vi "PH_Tektronix_7000.ProcCases.vi"(0 "i ref in":refnum<vi>, 1 "selector":string, 2 "Data":T4, 3 "call cluster":T5={"Object"="", "Selector"="", "CallType"=enum."synchronous", "Async Object"="", "Async Selector"="", "Data Descriptor"="", "Data"=[], "Error #"=0, "Expire"=0}, 5 "error in (no error)":errorcluster) -> (14 "i ref out":refnum<vi>, 17 "answer cluster":T5={"Object"="", "Selector"="", "CallType"=enum."synchronous", "Async Object"="", "Async Selector"="", "Data Descriptor"="", "Data"=[], "Error #"=0, "Expire"=0}, 19 "error out":errorcluster)   [LabVIEW 2014, in "PH_Tektronix_7000.lvlib"]
doc: "This method is called by a process from within the default case in the event loop. The methods of a class that are linked to events will be called from THIS method. Add your code here."
uses:
  PH_Tektronix_7000.lvlib
  CSCore/CSSystem/CoreDefs/CoreDefs.call_type.ctl
  CSCore/BaseProcess/BaseProcess.descriptor string definition.ctl
  CSCore/CSSystem/CoreDefs/CoreDefs.rawDataType.ctl
  PH_Tektronix_7000.Channel Config.ctl
  PH_Tektronix_7000.Trigger Config.ctl
  PH_Tektronix_7000.Acquisition Config.ctl
  CSCore/CSSystem/CoreLib/CoreLib.string 2 byte array.vi
  CSCore/CSSystem/CoreLib/CoreLib.byte array 2 short.vi
  CSCore/CSSystem/CoreLib/CoreLib.byte array 2 double.vi
  CSCore/CSSystem/CoreLib/CoreLib.byte array 2 string.vi
  CSCore/CSSystem/CoreLib/CoreLib.byte array 2 int.vi
  CSCore/BaseProcess/BaseProcess.lvlib
  CSCore/CSSystem/CoreLib/CoreLib.lvlib
  PH_PSDBWriter/PH_PSDBWriter.lvlib
  CSCore/CAEObj/CAEObj.lvlib
  CSCore/CSSystem/CSSystemLib/CSSystemLib.lvlib
panel:
  in  "Acqu Config":T1={"Record Length"=0, "Timebase [s/div]"=10000.0, "Position [%]"=0.0, "Acquisition Type"=1, "Average Waveforms"=10, "Envelope Waveforms"=10, "WfmDB Samples"=16000, "Continuous?"=FALSE, "Delay [s]"=0.0, "Run?"=FALSE} {"Delay [s]" format="%#_12p"; "Acquisition Type" items=["Sample", "Peak Detect", "Hi Res", "Average", "Envelope", "WfmDB"]; "Timebase [s/div]" format="%#_12g"}
  in  "Trig Config":T2 {"Trigger Mode" items=["Normal", "Auto"]; "Coupling" items=["DC", "AC", "Hf Reject", "Lf Reject", "Noise Rej", "Atrigger"]; "Slope" items=["Rise", "Fall", "Either"]; "Source" items=["Channel1"=0, "Channel2"=1, "Channel3"=2, "Channel4"=3, "Aux"=12, "Line"=13]}
  in  "Channel Config":T3={"Enable Channel"=FALSE, "Bandwidth"=0, "Input Impedance"=0, "Vertical Coupling"=0, "Probe Attenuation"=1.0, "Range [V/div]"=1.0, "Position [div]"=10.0, "Bandwidth raw"=""} {"Vertical Coupling" items=["AC", "DC", "Ground"]; "Input Impedance" items=["1M", "50"]; "Bandwidth" items=["FULL", "500 MHz", "250 MHz", "150 MHz", "20 MHz"]}
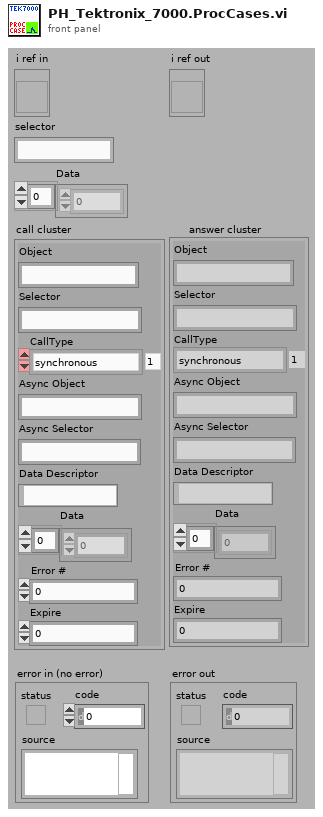
[diagram p1: front panel]
types:
  T1 = typedef "PH_Tektronix_7000.lvlib/PH_Tektronix_7000.Acquisition Config.ctl" = cluster{"Record Length":u32, "Timebase [s/div]":dbl, "Position [%]":dbl, "Acquisition Type":u16, "Average Waveforms":i32, "Envelope Waveforms":i32, "WfmDB Samples":i32, "Continuous?":bool, "Delay [s]":dbl, "Run?":bool}
  T2 = typedef "PH_Tektronix_7000.lvlib/PH_Tektronix_7000.Trigger Config.ctl" = cluster{"Source":u16, "Level [V]":dbl, "Slope":u16, "Coupling":u16, "Trigger Mode":u16}
  T3 = typedef "PH_Tektronix_7000.lvlib/PH_Tektronix_7000.Channel Config.ctl" = cluster{"Enable Channel":bool, "Bandwidth":u16, "Input Impedance":u16, "Vertical Coupling":u16, "Probe Attenuation":dbl, "Range [V/div]":dbl, "Position [div]":dbl, "Bandwidth raw":string}
  T4 = typedef "CoreDefs.rawDataType.ctl" = i8[]
  T5 = typedef "CoreDefs.call_type.ctl" = cluster{"Object":string, "Selector":string, "CallType":enum16{"simple", "synchronous", "asynchronous"}, "Async Object":string, "Async Selector":string, "Data Descriptor":T6, "Data":T4, "Error #":i32, "Expire":u32}
  T6 = typedef "BaseProcess.lvlib/BaseProcess.descriptor string definition.ctl" = string
  T7 = typedef "PH_PSDBWriter.lvlib/PH_PSDBWriter.PHELIX-Subsystems.ctl" = i32
  T8 = typedef "PH_Tektronix_7000.lvlib/PH_Tektronix_7000.i attribute.ctl" = cluster{"VISA Resource Name":refnum<visa-resource-name>, "IDN":cluster{"Instrument Driver":string, "Instrument Firmware":string, "Model":string, "Serial Number":string}, "Selftest":cluster{"Result":i32, "Message":string}, "Trigger Configuration":T2, "Acquisition Configuration":T1, "GUI Refs":T9, "State":T10, "Error Message":string, "Allow Prdc Loop?":bool, "Channel 1":T3, "Channel 2":T3, "Channel 3":T3, "Channel 4":T3, "Data CH 1":waveform(dbl), "Data CH 2":waveform(dbl), "Data CH 3":waveform(dbl), "Data CH 4":waveform(dbl), "Allow config?":bool, "Name Channel 1":string, "Name Channel 2":string, "Name Channel 3":string, "Name Channel 4":string, "Fetch Data before sending to PSDB?":bool, "Constructor passed?":bool, "Data taken at":timestamp, "Plot Colors":u32[], "Default VISA Resource":string}
  T9 = typedef "PH_Tektronix_7000.lvlib/PH_Tektronix_7000.GUI Refs.ctl" = cluster{"Graph":refnum<vi>, "State":refnum<vi>, "Delete":refnum<vi>, "VISA Resource":refnum<vi>, "Allow Configure":refnum<vi>, "Fetch Data":refnum<vi>, "Fetch before sending Data to PSDB":refnum<vi>, "Name Channel 1":refnum<vi>, "Name Channel 2":refnum<vi>, "Name Channel 3":refnum<vi>, "Name Channel 4":refnum<vi>, "Prdc Intervall [ms]":refnum<vi>, "Data taken":refnum<vi>, "Model":refnum<vi>, "Serial Number":refnum<vi>, "Firmware":refnum<vi>, "Driver":refnum<vi>, "Acquisition":refnum<vi>, "Trigger":refnum<vi>, "Cursor: D Time [s]":refnum<vi>, "Cursor: D Signal [V]":refnum<vi>, "Channel 1":refnum<vi>, "Channel 2":refnum<vi>, "Channel 3":refnum<vi>, "Channel 4":refnum<vi>}
  T10 = typedef "PH_StatusHandler.lvlib/PH_StatusHandler.Status.ctl" = i16
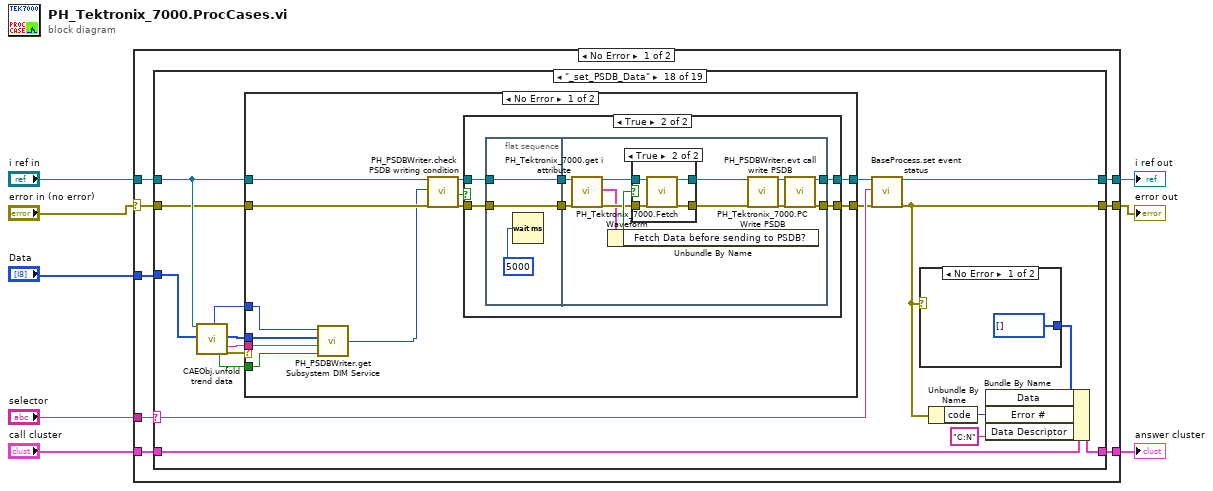
[diagram p0: block diagram]
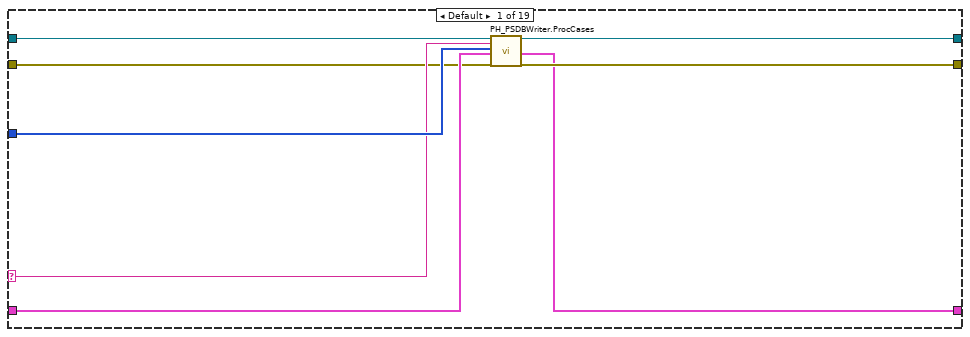
[diagram p2: hidden frame]
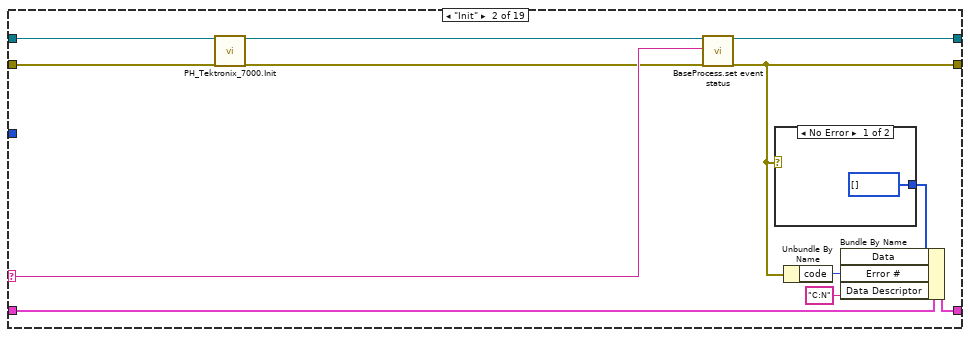
[diagram p3: hidden frame]
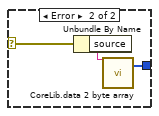
[diagram p4: hidden frame]
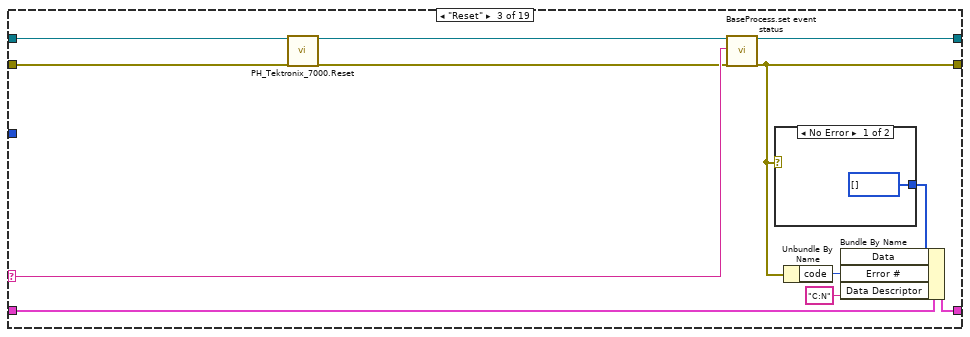
[diagram p5: hidden frame]
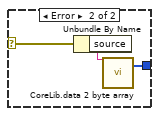
[diagram p6: hidden frame]
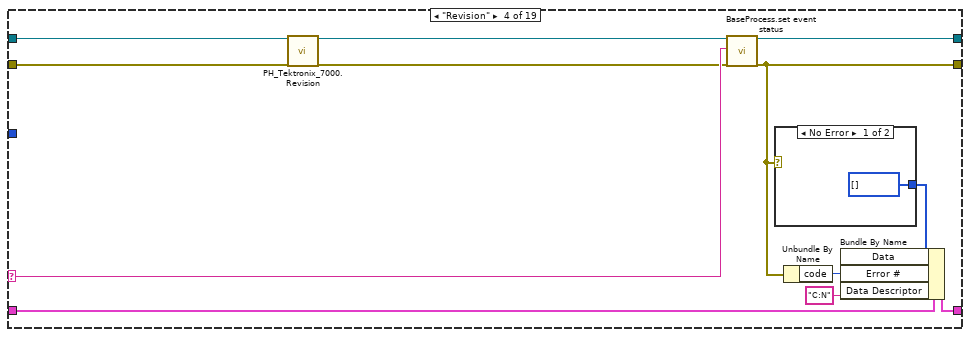
[diagram p7: hidden frame]
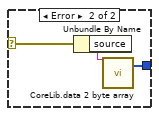
[diagram p8: hidden frame]
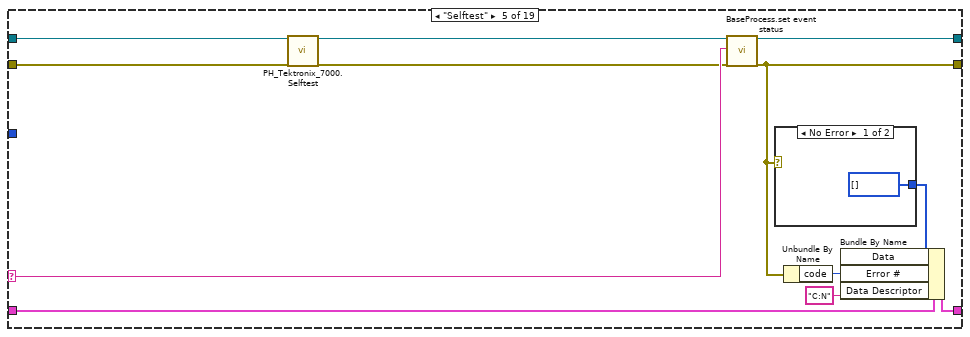
[diagram p9: hidden frame]
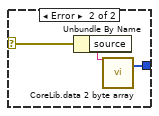
[diagram p10: hidden frame]
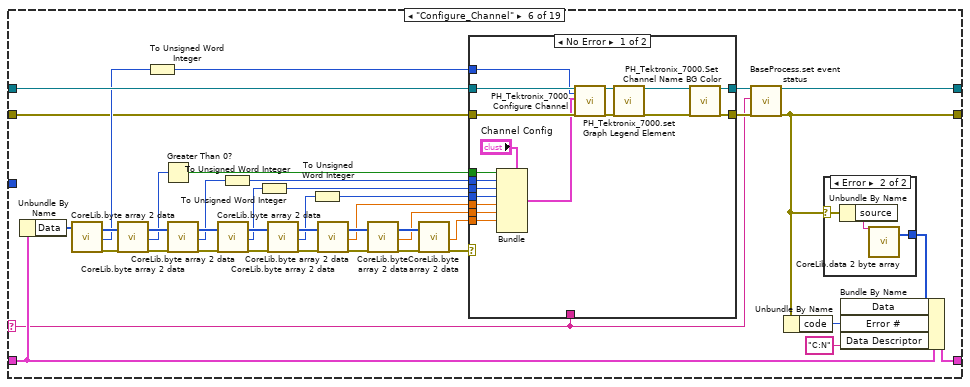
[diagram p11: hidden frame]
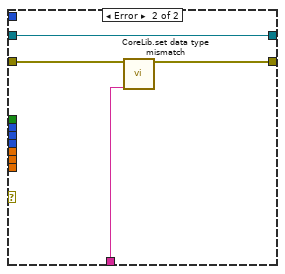
[diagram p12: hidden frame]
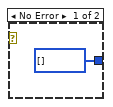
[diagram p13: hidden frame]
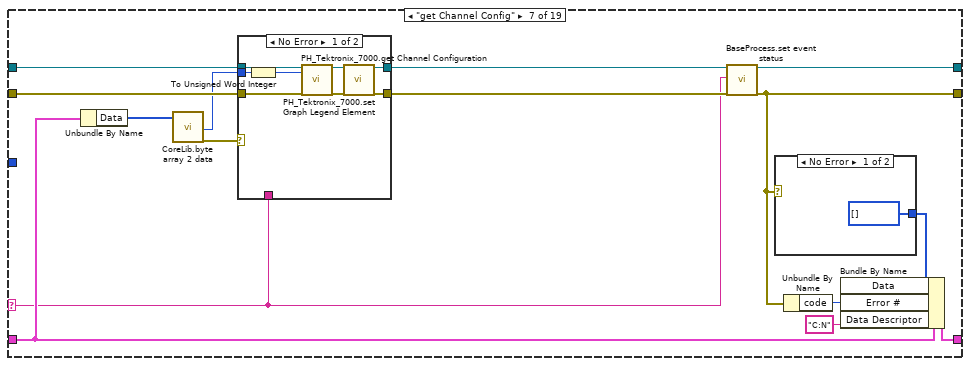
[diagram p14: hidden frame]
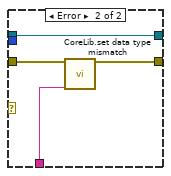
[diagram p15: hidden frame]
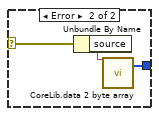
[diagram p16: hidden frame]
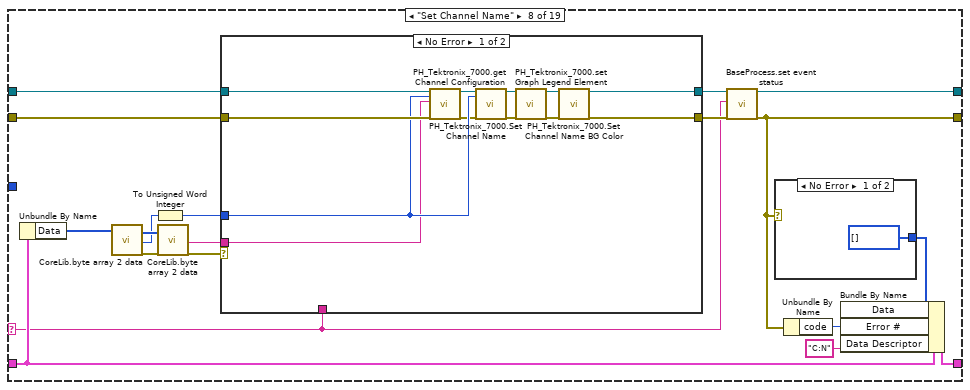
[diagram p17: hidden frame]
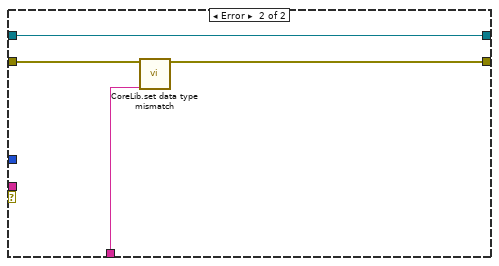
[diagram p18: hidden frame]
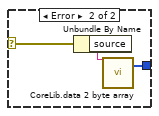
[diagram p19: hidden frame]
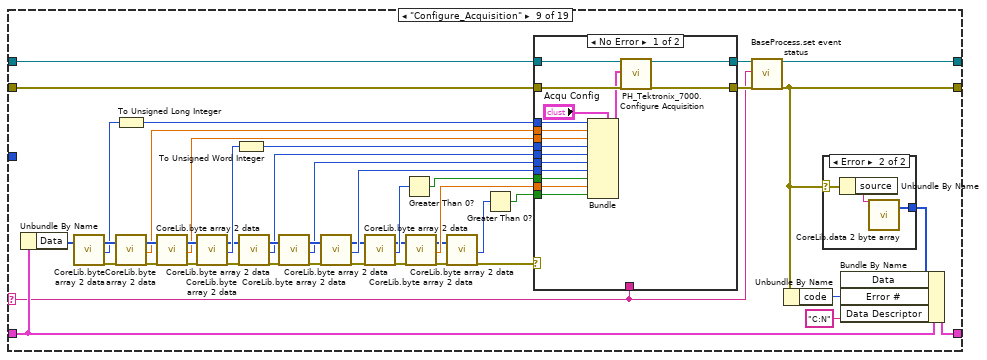
[diagram p20: hidden frame]
diagram:
  n1 = case shown="No Error" "error in (no error)" {
    selector: "error in (no error)" -> [w9 w614]
    tunnel: "selector" -> [w16 _]
    tunnel: [w15 w615] -> w7
    tunnel: "Data" -> [w14 _]
    tunnel: "call cluster" -> [w13 w615]
    tunnel: "i ref in" -> [w12 w616]
    tunnel: [w11 w616] -> w3
    tunnel: [w10 w614] -> w2
    frame No Error {
      n2 = case shown="\"_set_PSDB_Data\"" w16 {
        selector: w16 -> [w19 w29 w45 w61 w77 w100 w156 w192 w252 w297 w324 w363 w379 w394 w423 w464 w494 w543 w602]
        tunnel: w14 -> [w20 _ _ _ _ _ _ _ _ _ _ _ _ _ _ _ _ w533 _]
        tunnel: w12 -> [w18 w28 w44 w60 w76 w123 w164 w199 w265 w301 w336 w367 w383 w400 w429 w470 w499 w537 w601]
        tunnel: [w24 w32 w48 w64 w80 w125 w166 w201 w267 w303 w338 w369 w385 w405 w434 w475 w503 w546 w605] -> w11
        tunnel: w13 -> [w21 w30 w46 w62 w78 w120 w159 w196 w261 w298 w332 w364 w380 w398 w427 w468 w497 w544 w603]
        tunnel: [w22 w35 w51 w67 w83 w128 w169 w204 w270 w306 w341 w372 w388 w408 w437 w478 w506 w549 w608] -> w15
        tunnel: w9 -> [w17 w27 w43 w59 w75 w98 w161 w191 w251 w296 w323 w362 w378 w397 w426 w467 w496 w536 w599]
        tunnel: [w23 w33 w49 w65 w81 w126 w167 w202 w268 w304 w339 w370 w386 w406 w435 w476 w504 w547 w606] -> w10
        frame Default {
          n3 = call "PH_PSDBWriter.ProcCases.vi"("i ref in"=w18, "selector"=w19, "Data"=w20, "call cluster"=w21, "error in"=w17) -> ("i ref out"=w24:refnum<vi>, "answer cluster"=w22:T5, "error out"=w23:errorcluster)  [unwired: 12 in]
        }
        frame "Init" {
          n4 = call "PH_Tektronix_7000.Init.vi"("i ref in"=w28, "error in (no error)"=w27) -> ("i ref out"=w26:refnum<vi>, "error out"=w25:errorcluster)  [unwired: 16 in]
          n5 = call "BaseProcess.set event status.vi"("i ref in"=w26, "EventStatus"=w29, "error in (no error)"=w25) -> ("i ref out"=w32:refnum<vi>, "error out"=w33:errorcluster)  [unwired: 14 in, 1 out]
          n6 = case shown="No Error" w33 {
            selector: w33 -> [_ w40]
            tunnel: [T4 [] ("byteArray out") w39] -> w34
            frame No Error {
            }
            frame Error {
              n7 = Unbundle By Name(w40) -> ("source"=w38:string)
              n8 = call-poly "CoreLib.data 2 byte array.vi"("string"=w38) -> ("byteArray out"=w39:T4)  [unwired: 18 in]
            }
          }
          n9 = Unbundle By Name(w33) -> ("code"=w36:i32)
          n10 = Bundle By Name(cluster=w30, "Data"=w34, "Error #"=w36, "Data Descriptor"="C:N") -> (w35:T5)
        }
        frame "Reset" {
          n11 = call "PH_Tektronix_7000.Reset.vi"("i ref in"=w44, "error IO"=w43) -> ("i ref out"=w41:refnum<vi>, "error out"=w42:errorcluster)  [unwired: 16 in]
          n12 = call "BaseProcess.set event status.vi"("i ref in"=w41, "EventStatus"=w45, "error in (no error)"=w42) -> ("i ref out"=w48:refnum<vi>, "error out"=w49:errorcluster)  [unwired: 14 in, 1 out]
          n13 = case shown="No Error" w49 {
            selector: w49 -> [_ w56]
            tunnel: [T4 [] ("byteArray out") w55] -> w50
            frame No Error {
            }
            frame Error {
              n14 = Unbundle By Name(w56) -> ("source"=w54:string)
              n15 = call-poly "CoreLib.data 2 byte array.vi"("string"=w54) -> ("byteArray out"=w55:T4)  [unwired: 18 in]
            }
          }
          n16 = Unbundle By Name(w49) -> ("code"=w52:i32)
          n17 = Bundle By Name(cluster=w46, "Data"=w50, "Error #"=w52, "Data Descriptor"="C:N") -> (w51:T5)
        }
        frame "Revision" {
          n18 = call "PH_Tektronix_7000.Revision.vi"("i ref in"=w60, "error IO"=w59) -> ("i ref out"=w57:refnum<vi>, "error out"=w58:errorcluster)  [unwired: 16 in]
          n19 = call "BaseProcess.set event status.vi"("i ref in"=w57, "EventStatus"=w61, "error in (no error)"=w58) -> ("i ref out"=w64:refnum<vi>, "error out"=w65:errorcluster)  [unwired: 14 in, 1 out]
          n20 = case shown="No Error" w65 {
            selector: w65 -> [_ w72]
            tunnel: [T4 [] ("byteArray out") w71] -> w66
            frame No Error {
            }
            frame Error {
              n21 = Unbundle By Name(w72) -> ("source"=w70:string)
              n22 = call-poly "CoreLib.data 2 byte array.vi"("string"=w70) -> ("byteArray out"=w71:T4)  [unwired: 18 in]
            }
          }
          n23 = Unbundle By Name(w65) -> ("code"=w68:i32)
          n24 = Bundle By Name(cluster=w62, "Data"=w66, "Error #"=w68, "Data Descriptor"="C:N") -> (w67:T5)
        }
        frame "Selftest" {
          n25 = call "PH_Tektronix_7000.Selftest.vi"("i ref in"=w76, "error IO"=w75) -> ("i ref out"=w73:refnum<vi>, "error out"=w74:errorcluster)  [unwired: 16 in]
          n26 = call "BaseProcess.set event status.vi"("i ref in"=w73, "EventStatus"=w77, "error in (no error)"=w74) -> ("i ref out"=w80:refnum<vi>, "error out"=w81:errorcluster)  [unwired: 14 in, 1 out]
          n27 = case shown="No Error" w81 {
            selector: w81 -> [_ w88]
            tunnel: [T4 [] ("byteArray out") w87] -> w82
            frame No Error {
            }
            frame Error {
              n28 = Unbundle By Name(w88) -> ("source"=w86:string)
              n29 = call-poly "CoreLib.data 2 byte array.vi"("string"=w86) -> ("byteArray out"=w87:T4)  [unwired: 18 in]
            }
          }
          n30 = Unbundle By Name(w81) -> ("code"=w84:i32)
          n31 = Bundle By Name(cluster=w78, "Data"=w82, "Error #"=w84, "Data Descriptor"="C:N") -> (w83:T5)
        }
        frame "Configure_Channel" {
          n32 = Unbundle By Name(w120) -> ("Data"=w90:T4)
          n33 = call-poly "CoreLib.byte array 2 data.vi"("byteArray"=w90) -> ("byteArray out"=w112:T4, "i16"=w105:i16, "error out"=w119:errorcluster)  [unwired: 16 in]
          n34 = call-poly "CoreLib.byte array 2 data.vi"("byteArray"=w112, "error in (no error)"=w119) -> ("byteArray out"=w111:T4, "i16"=w95:i16, "error out"=w118:errorcluster)  [unwired: 15 in]
          n35 = To Unsigned Word Integer(number=w105) -> (unsigned 16bit integer=w89:u16)
          n36 = Greater Than 0?(x=w95) -> (x > 0?=w94:bool)
          n37 = call-poly "CoreLib.byte array 2 data.vi"("byteArray"=w111, "error in (no error)"=w118) -> ("byteArray out"=w110:T4, "i16"=w104:i16, "error out"=w117:errorcluster)  [unwired: 15 in]
          n38 = call-poly "CoreLib.byte array 2 data.vi"("byteArray"=w110, "error in (no error)"=w117) -> ("byteArray out"=w109:T4, "i16"=w97:i16, "error out"=w116:errorcluster)  [unwired: 15 in]
          n39 = To Unsigned Word Integer(number=w104) -> (unsigned 16bit integer=w93:u16)
          n40 = To Unsigned Word Integer(number=w97) -> (unsigned 16bit integer=w92:u16)
          n41 = call-poly "CoreLib.byte array 2 data.vi"("byteArray"=w109, "error in (no error)"=w116) -> ("byteArray out"=w108:T4, "i16"=w96:i16, "error out"=w115:errorcluster)  [unwired: 15 in]
          n42 = To Unsigned Word Integer(number=w96) -> (unsigned 16bit integer=w91:u16)
          n43 = call-poly "CoreLib.byte array 2 data.vi"("byteArray"=w108, "error in (no error)"=w115) -> ("byteArray out"=w107:T4, "d64"=w103:dbl, "error out"=w114:errorcluster)  [unwired: 15 in]
          n44 = call-poly "CoreLib.byte array 2 data.vi"("byteArray"=w107, "error in (no error)"=w114) -> ("byteArray out"=w106:T4, "d64"=w102:dbl, "error out"=w113:errorcluster)  [unwired: 15 in]
          n45 = call-poly "CoreLib.byte array 2 data.vi"("byteArray"=w106, "error in (no error)"=w113) -> ("d64"=w101:dbl, "error out"=w99:errorcluster)  [unwired: 15 in, 1 out]
          n46 = case shown="No Error" w99 {
            tunnel: w123 -> [w147 w151]
            tunnel: [w132 w149] -> w122
            tunnel: [w130 w151] -> w121
            tunnel: w94 -> [w143 _]
            tunnel: w93 -> [w142 _]
            tunnel: w92 -> [w141 _]
            tunnel: w91 -> [w140 _]
            tunnel: w103 -> [w139 _]
            tunnel: w102 -> [w138 _]
            tunnel: w101 -> [w137 _]
            tunnel: w100 -> [_ w150]
            tunnel: w98 -> [w146 w148]
            tunnel: w89 -> [w136 _]
            frame No Error {
              n47 = Bundle(cluster="Channel Config", "Enable Channel"=w143, "Bandwidth"=w142, "Input Impedance"=w141, "Vertical Coupling"=w140, "Probe Attenuation"=w139, "Range [V/div]"=w138, "Position [div]"=w137) -> (w144:T3)  [unwired: 1 in]
              n48 = call "PH_Tektronix_7000.Configure Channel.vi"("i ref in"=w147, "Channel"=w136, "Channel Configuration"=w144, "error IO"=w146) -> ("i ref out"=w133:refnum<vi>, "error out"=w134:errorcluster)  [unwired: 14 in]
              n49 = call "PH_Tektronix_7000.set Graph Legend Element.vi"("i ref in"=w133, "error in (no error)"=w134) -> ("i ref out"=w131:refnum<vi>, "error out"=w135:errorcluster)  [unwired: 16 in]
              n50 = call "PH_Tektronix_7000.Set Channel Name BG Color.vi"("i ref in"=w131, "error in"=w135) -> ("i ref out"=w130:refnum<vi>, "error out"=w132:errorcluster)  [unwired: 16 in]
            }
            frame Error {
              n51 = call "CoreLib.set data type mismatch.vi"("error in (no error)"=w148, "error source"=w150) -> ("error out"=w149:errorcluster)  [unwired: 17 in]
            }
          }
          n52 = call "BaseProcess.set event status.vi"("i ref in"=w121, "EventStatus"=w100, "error in (no error)"=w122) -> ("i ref out"=w125:refnum<vi>, "error out"=w126:errorcluster)  [unwired: 14 in, 1 out]
          n53 = Unbundle By Name(w126) -> ("code"=w129:i32)
          n54 = case shown="Error" w126 {
            selector: w126 -> [_ w155]
            tunnel: [T4 [] ("byteArray out") w154] -> w127
            frame No Error {
            }
            frame Error {
              n55 = Unbundle By Name(w155) -> ("source"=w153:string)
              n56 = call-poly "CoreLib.data 2 byte array.vi"("string"=w153) -> ("byteArray out"=w154:T4)  [unwired: 18 in]
            }
          }
          n57 = Bundle By Name(cluster=w120, "Data"=w127, "Error #"=w129, "Data Descriptor"="C:N") -> (w128:T5)
        }
        frame "get Channel Config" {
          n58 = Unbundle By Name(w159) -> ("Data"=w160:T4)
          n59 = call-poly "CoreLib.byte array 2 data.vi"("byteArray"=w160) -> ("i16"=w158:i16, "error out"=w157:errorcluster)  [unwired: 16 in, 1 out]
          n60 = case shown="No Error" w157 {
            tunnel: w164 -> [w178 w180]
            tunnel: [w171 w181] -> w163
            tunnel: [w173 w180] -> w162
            tunnel: w161 -> [w177 w182]
            tunnel: w158 -> [w175 _]
            tunnel: w156 -> [_ w179]
            frame No Error {
              n61 = To Unsigned Word Integer(number=w175) -> (unsigned 16bit integer=w176:u16)
              n62 = call "PH_Tektronix_7000.get Channel Configuration.vi"("i ref in"=w178, "Channel"=w176, "error IO"=w177) -> ("i ref out"=w174:refnum<vi>, "error out"=w172:errorcluster)  [unwired: 15 in]
              n63 = call "PH_Tektronix_7000.set Graph Legend Element.vi"("i ref in"=w174, "error in (no error)"=w172) -> ("i ref out"=w173:refnum<vi>, "error out"=w171:errorcluster)  [unwired: 16 in]
            }
            frame Error {
              n64 = call "CoreLib.set data type mismatch.vi"("error in (no error)"=w182, "error source"=w179) -> ("error out"=w181:errorcluster)  [unwired: 17 in]
            }
          }
          n65 = call "BaseProcess.set event status.vi"("i ref in"=w162, "EventStatus"=w156, "error in (no error)"=w163) -> ("i ref out"=w166:refnum<vi>, "error out"=w167:errorcluster)  [unwired: 14 in, 1 out]
          n66 = case shown="No Error" w167 {
            selector: w167 -> [_ w186]
            tunnel: [T4 [] ("byteArray out") w185] -> w168
            frame No Error {
            }
            frame Error {
              n67 = Unbundle By Name(w186) -> ("source"=w184:string)
              n68 = call-poly "CoreLib.data 2 byte array.vi"("string"=w184) -> ("byteArray out"=w185:T4)  [unwired: 18 in]
            }
          }
          n69 = Unbundle By Name(w167) -> ("code"=w170:i32)
          n70 = Bundle By Name(cluster=w159, "Data"=w168, "Error #"=w170, "Data Descriptor"="C:N") -> (w169:T5)
        }
        frame "Set Channel Name" {
          n71 = Unbundle By Name(w196) -> ("Data"=w190:T4)
          n72 = call-poly "CoreLib.byte array 2 data.vi"("byteArray"=w190) -> ("byteArray out"=w194:T4, "i16"=w193:i16, "error out"=w195:errorcluster)  [unwired: 16 in]
          n73 = To Unsigned Word Integer(number=w193) -> (unsigned 16bit integer=w189:u16)
          n74 = call-poly "CoreLib.byte array 2 data.vi"("byteArray"=w194, "error in (no error)"=w195) -> ("string"=w188:string, "error out"=w187:errorcluster)  [unwired: 15 in, 1 out]
          n75 = case shown="No Error" w187 {
            tunnel: w199 -> [w217 w221]
            tunnel: [w208 w219] -> w198
            tunnel: [w206 w221] -> w197
            tunnel: w192 -> [_ w220]
            tunnel: w191 -> [w216 w218]
            tunnel: w189 -> [w212 _]
            tunnel: w188 -> [w209 _]
            frame No Error {
              n76 = call "PH_Tektronix_7000.Set Channel Name.vi"("i ref in"=w217, "Channel"=w212, "Channel Name"=w209, "error IO"=w216) -> ("i ref out"=w211:refnum<vi>, "error out"=w210:errorcluster)  [unwired: 14 in]
              n77 = call "PH_Tektronix_7000.get Channel Configuration.vi"("i ref in"=w211, "Channel"=w212, "error IO"=w210) -> ("i ref out"=w215:refnum<vi>, "error out"=w214:errorcluster)  [unwired: 15 in]
              n78 = call "PH_Tektronix_7000.set Graph Legend Element.vi"("i ref in"=w215, "error in (no error)"=w214) -> ("i ref out"=w207:refnum<vi>, "error out"=w213:errorcluster)  [unwired: 16 in]
              n79 = call "PH_Tektronix_7000.Set Channel Name BG Color.vi"("i ref in"=w207, "error in"=w213) -> ("i ref out"=w206:refnum<vi>, "error out"=w208:errorcluster)  [unwired: 16 in]
            }
            frame Error {
              n80 = call "CoreLib.set data type mismatch.vi"("error in (no error)"=w218, "error source"=w220) -> ("error out"=w219:errorcluster)  [unwired: 17 in]
            }
          }
          n81 = call "BaseProcess.set event status.vi"("i ref in"=w197, "EventStatus"=w192, "error in (no error)"=w198) -> ("i ref out"=w201:refnum<vi>, "error out"=w202:errorcluster)  [unwired: 14 in, 1 out]
          n82 = case shown="No Error" w202 {
            selector: w202 -> [_ w225]
            tunnel: [T4 [] ("byteArray out") w224] -> w203
            frame No Error {
            }
            frame Error {
              n83 = Unbundle By Name(w225) -> ("source"=w223:string)
              n84 = call-poly "CoreLib.data 2 byte array.vi"("string"=w223) -> ("byteArray out"=w224:T4)  [unwired: 18 in]
            }
          }
          n85 = Unbundle By Name(w202) -> ("code"=w205:i32)
          n86 = Bundle By Name(cluster=w196, "Data"=w203, "Error #"=w205, "Data Descriptor"="C:N") -> (w204:T5)
        }
        frame "Configure_Acquisition" {
          n87 = Unbundle By Name(w261) -> ("Data"=w262:T4)
          n88 = call-poly "CoreLib.byte array 2 data.vi"("byteArray"=w262) -> ("byteArray out"=w257:T4, "i32"=w254:i32, "error out"=w260:errorcluster)  [unwired: 16 in]
          n89 = To Unsigned Long Integer(number=w254) -> (unsigned 32bit integer=w247:u32)
          n90 = call-poly "CoreLib.byte array 2 data.vi"("byteArray"=w257, "error in (no error)"=w260) -> ("byteArray out"=w256:T4, "d64"=w246:dbl, "error out"=w259:errorcluster)  [unwired: 15 in]
          n91 = call-poly "CoreLib.byte array 2 data.vi"("byteArray"=w256, "error in (no error)"=w259) -> ("byteArray out"=w255:T4, "d64"=w253:dbl, "error out"=w258:errorcluster)  [unwired: 15 in]
          n92 = call-poly "CoreLib.byte array 2 data.vi"("byteArray"=w255, "error in (no error)"=w258) -> ("byteArray out"=w240:T4, "i16"=w248:i16, "error out"=w239:errorcluster)  [unwired: 15 in]
          n93 = To Unsigned Word Integer(number=w248) -> (unsigned 16bit integer=w245:u16)
          n94 = call-poly "CoreLib.byte array 2 data.vi"("byteArray"=w240, "error in (no error)"=w239) -> ("byteArray out"=w242:T4, "i32"=w238:i32, "error out"=w244:errorcluster)  [unwired: 15 in]
          n95 = call-poly "CoreLib.byte array 2 data.vi"("byteArray"=w242, "error in (no error)"=w244) -> ("byteArray out"=w241:T4, "i32"=w237:i32, "error out"=w243:errorcluster)  [unwired: 15 in]
          n96 = call-poly "CoreLib.byte array 2 data.vi"("byteArray"=w241, "error in (no error)"=w243) -> ("byteArray out"=w226:T4, "i32"=w236:i32, "error out"=w229:errorcluster)  [unwired: 15 in]
          n97 = call-poly "CoreLib.byte array 2 data.vi"("byteArray"=w226, "error in (no error)"=w229) -> ("byteArray out"=w234:T4, "i16"=w250:i16, "error out"=w235:errorcluster)  [unwired: 15 in]
          n98 = Greater Than 0?(x=w250) -> (x > 0?=w249:bool)
          n99 = call-poly "CoreLib.byte array 2 data.vi"("byteArray"=w234, "error in (no error)"=w235) -> ("byteArray out"=w230:T4, "d64"=w233:dbl, "error out"=w232:errorcluster)  [unwired: 15 in]
          n100 = call-poly "CoreLib.byte array 2 data.vi"("byteArray"=w230, "error in (no error)"=w232) -> ("i16"=w228:i16, "error out"=w231:errorcluster)  [unwired: 15 in, 1 out]
          n101 = Greater Than 0?(x=w228) -> (x > 0?=w227:bool)
          n102 = case shown="No Error" w231 {
            tunnel: w265 -> [w287 w291]
            tunnel: [w272 w289] -> w264
            tunnel: [w273 w291] -> w263
            tunnel: w247 -> [w284 _]
            tunnel: w246 -> [w283 _]
            tunnel: w253 -> [w282 _]
            tunnel: w245 -> [w281 _]
            tunnel: w249 -> [w276 _]
            tunnel: w252 -> [_ w290]
            tunnel: w251 -> [w286 w288]
            tunnel: w238 -> [w279 _]
            tunnel: w237 -> [w278 _]
            tunnel: w236 -> [w277 _]
            tunnel: w233 -> [w275 _]
            tunnel: w227 -> [w274 _]
            frame No Error {
              n103 = Bundle(cluster="Acqu Config", "Record Length"=w284, "Timebase [s/div]"=w283, "Position [%]"=w282, "Acquisition Type"=w281, "Average Waveforms"=w279, "Envelope Waveforms"=w278, "WfmDB Samples"=w277, "Continuous?"=w276, "Delay [s]"=w275, "Run?"=w274) -> (w280:T1)
              n104 = call "PH_Tektronix_7000.Configure Acquisition.vi"("i ref in"=w287, "Acquisition Configuration"=w280, "error IO"=w286) -> ("i ref out"=w273:refnum<vi>, "error out"=w272:errorcluster)  [unwired: 15 in]
            }
            frame Error {
              n105 = call "CoreLib.set data type mismatch.vi"("error in (no error)"=w288, "error source"=w290) -> ("error out"=w289:errorcluster)  [unwired: 17 in]
            }
          }
          n106 = call "BaseProcess.set event status.vi"("i ref in"=w263, "EventStatus"=w252, "error in (no error)"=w264) -> ("i ref out"=w267:refnum<vi>, "error out"=w268:errorcluster)  [unwired: 14 in, 1 out]
          n107 = Unbundle By Name(w268) -> ("code"=w271:i32)
          n108 = case shown="Error" w268 {
            selector: w268 -> [_ w295]
            tunnel: [T4 [] ("byteArray out") w294] -> w269
            frame No Error {
            }
            frame Error {
              n109 = Unbundle By Name(w295) -> ("source"=w293:string)
              n110 = call-poly "CoreLib.data 2 byte array.vi"("string"=w293) -> ("byteArray out"=w294:T4)  [unwired: 18 in]
            }
          }
          n111 = Bundle By Name(cluster=w261, "Data"=w269, "Error #"=w271, "Data Descriptor"="C:N") -> (w270:T5)
        }
        frame "get Acquisition Config" {
          n112 = call "PH_Tektronix_7000.get Acquisition Configuration.vi"("i ref in"=w301, "error IO"=w296) -> ("i ref out"=w299:refnum<vi>, "error out"=w300:errorcluster)  [unwired: 16 in]
          n113 = call "BaseProcess.set event status.vi"("i ref in"=w299, "EventStatus"=w297, "error in (no error)"=w300) -> ("i ref out"=w303:refnum<vi>, "error out"=w304:errorcluster)  [unwired: 14 in, 1 out]
          n114 = case shown="No Error" w304 {
            selector: w304 -> [_ w311]
            tunnel: [T4 [] ("byteArray out") w310] -> w305
            frame No Error {
            }
            frame Error {
              n115 = Unbundle By Name(w311) -> ("source"=w309:string)
              n116 = call-poly "CoreLib.data 2 byte array.vi"("string"=w309) -> ("byteArray out"=w310:T4)  [unwired: 18 in]
            }
          }
          n117 = Unbundle By Name(w304) -> ("code"=w307:i32)
          n118 = Bundle By Name(cluster=w298, "Data"=w305, "Error #"=w307, "Data Descriptor"="C:N") -> (w306:T5)
        }
        frame "Configure_Trigger" {
          n119 = Unbundle By Name(w332) -> ("Data"=w333:T4)
          n120 = call-poly "CoreLib.byte array 2 data.vi"("byteArray"=w333) -> ("byteArray out"=w329:T4, "i16"=w327:i16, "error out"=w331:errorcluster)  [unwired: 16 in]
          n121 = call-poly "CoreLib.byte array 2 data.vi"("byteArray"=w329, "error in (no error)"=w331) -> ("byteArray out"=w328:T4, "d64"=w326:dbl, "error out"=w330:errorcluster)  [unwired: 15 in]
          n122 = call-poly "CoreLib.byte array 2 data.vi"("byteArray"=w328, "error in (no error)"=w330) -> ("byteArray out"=w317:T4, "i16"=w325:i16, "error out"=w322:errorcluster)  [unwired: 15 in]
          n123 = call-poly "CoreLib.byte array 2 data.vi"("byteArray"=w317, "error in (no error)"=w322) -> ("byteArray out"=w314:T4, "i16"=w321:i16, "error out"=w316:errorcluster)  [unwired: 15 in]
          n124 = call-poly "CoreLib.byte array 2 data.vi"("byteArray"=w314, "error in (no error)"=w316) -> ("i16"=w313:i16, "error out"=w315:errorcluster)  [unwired: 15 in, 1 out]
          n125 = To Unsigned Word Integer(number=w327) -> (unsigned 16bit integer=w320:u16)
          n126 = To Unsigned Word Integer(number=w325) -> (unsigned 16bit integer=w319:u16)
          n127 = To Unsigned Word Integer(number=w321) -> (unsigned 16bit integer=w318:u16)
          n128 = To Unsigned Word Integer(number=w313) -> (unsigned 16bit integer=w312:u16)
          n129 = case shown="No Error" w315 {
            tunnel: w336 -> [w353 w357]
            tunnel: [w343 w355] -> w335
            tunnel: [w344 w357] -> w334
            tunnel: w320 -> [w350 _]
            tunnel: w326 -> [w349 _]
            tunnel: w319 -> [w348 _]
            tunnel: w324 -> [_ w356]
            tunnel: w323 -> [w352 w354]
            tunnel: w318 -> [w346 _]
            tunnel: w312 -> [w345 _]
            frame No Error {
              n130 = Bundle(cluster="Trig Config", "Source"=w350, "Level [V]"=w349, "Slope"=w348, "Coupling"=w346, "Trigger Mode"=w345) -> (w347:T2)
              n131 = call "PH_Tektronix_7000.Configure Trigger.vi"("i ref in"=w353, "Trigger Configuration"=w347, "error IO"=w352) -> ("i ref out"=w344:refnum<vi>, "error out"=w343:errorcluster)  [unwired: 15 in]
            }
            frame Error {
              n132 = call "CoreLib.set data type mismatch.vi"("error in (no error)"=w354, "error source"=w356) -> ("error out"=w355:errorcluster)  [unwired: 17 in]
            }
          }
          n133 = call "BaseProcess.set event status.vi"("i ref in"=w334, "EventStatus"=w324, "error in (no error)"=w335) -> ("i ref out"=w338:refnum<vi>, "error out"=w339:errorcluster)  [unwired: 14 in, 1 out]
          n134 = case shown="No Error" w339 {
            selector: w339 -> [_ w361]
            tunnel: [T4 [] ("byteArray out") w360] -> w340
            frame No Error {
            }
            frame Error {
              n135 = Unbundle By Name(w361) -> ("source"=w359:string)
              n136 = call-poly "CoreLib.data 2 byte array.vi"("string"=w359) -> ("byteArray out"=w360:T4)  [unwired: 18 in]
            }
          }
          n137 = Unbundle By Name(w339) -> ("code"=w342:i32)
          n138 = Bundle By Name(cluster=w332, "Data"=w340, "Error #"=w342, "Data Descriptor"="C:N") -> (w341:T5)
        }
        frame "get Trigger Config" {
          n139 = call "PH_Tektronix_7000.get Trigger Configuration.vi"("i ref in"=w367, "error IO"=w362) -> ("i ref out"=w365:refnum<vi>, "error out"=w366:errorcluster)  [unwired: 16 in]
          n140 = call "BaseProcess.set event status.vi"("i ref in"=w365, "EventStatus"=w363, "error in (no error)"=w366) -> ("i ref out"=w369:refnum<vi>, "error out"=w370:errorcluster)  [unwired: 14 in, 1 out]
          n141 = case shown="No Error" w370 {
            selector: w370 -> [_ w377]
            tunnel: [T4 [] ("byteArray out") w376] -> w371
            frame No Error {
            }
            frame Error {
              n142 = Unbundle By Name(w377) -> ("source"=w375:string)
              n143 = call-poly "CoreLib.data 2 byte array.vi"("string"=w375) -> ("byteArray out"=w376:T4)  [unwired: 18 in]
            }
          }
          n144 = Unbundle By Name(w370) -> ("code"=w373:i32)
          n145 = Bundle By Name(cluster=w364, "Data"=w371, "Error #"=w373, "Data Descriptor"="C:N") -> (w372:T5)
        }
        frame "Fetch_Waveform" {
          n146 = call "PH_Tektronix_7000.Fetch Waveform.vi"("i ref in"=w383, "error IO"=w378) -> ("i ref out"=w381:refnum<vi>, "error out"=w382:errorcluster)  [unwired: 16 in]
          n147 = call "BaseProcess.set event status.vi"("i ref in"=w381, "EventStatus"=w379, "error in (no error)"=w382) -> ("i ref out"=w385:refnum<vi>, "error out"=w386:errorcluster)  [unwired: 14 in, 1 out]
          n148 = case shown="No Error" w386 {
            selector: w386 -> [_ w393]
            tunnel: [T4 [] ("byteArray out") w392] -> w387
            frame No Error {
            }
            frame Error {
              n149 = Unbundle By Name(w393) -> ("source"=w391:string)
              n150 = call-poly "CoreLib.data 2 byte array.vi"("string"=w391) -> ("byteArray out"=w392:T4)  [unwired: 18 in]
            }
          }
          n151 = Unbundle By Name(w386) -> ("code"=w389:i32)
          n152 = Bundle By Name(cluster=w380, "Data"=w387, "Error #"=w389, "Data Descriptor"="C:N") -> (w388:T5)
        }
        frame "Remote Control" {
          n153 = Unbundle By Name(w398) -> ("Data"=w402:T4)
          n154 = call-poly "CoreLib.byte array 2 data.vi"("byteArray"=w402) -> ("i16"=w403:i16, "error out"=w401:errorcluster)  [unwired: 16 in, 1 out]
          n155 = Greater Than 0?(x=w403) -> (x > 0?=w395:bool)
          n156 = case shown="No Error" w401 {
            tunnel: [w411 w418] -> w399
            tunnel: w400 -> [w413 w418]
            tunnel: w397 -> [w412 w417]
            tunnel: [w414 w416] -> w396
            tunnel: w394 -> [_ w415]
            tunnel: w395 -> [w410 _]
            frame No Error {
              n157 = call "PH_Tektronix_7000.PC Set Remote Control.vi"("i ref in"=w413, "Remote Controlled?"=w410, "error in (no error)"=w412) -> ("i ref out"=w411:refnum<vi>, "error out"=w414:errorcluster)  [unwired: 15 in]
            }
            frame Error {
              n158 = call "CoreLib.set data type mismatch.vi"("error in (no error)"=w417, "error source"=w415) -> ("error out"=w416:errorcluster)  [unwired: 17 in]
            }
          }
          n159 = call "BaseProcess.set event status.vi"("i ref in"=w399, "EventStatus"=w394, "error in (no error)"=w396) -> ("i ref out"=w405:refnum<vi>, "error out"=w406:errorcluster)  [unwired: 14 in, 1 out]
          n160 = case shown="No Error" w406 {
            selector: w406 -> [_ w422]
            tunnel: [T4 [] ("byteArray out") w421] -> w407
            frame No Error {
            }
            frame Error {
              n161 = Unbundle By Name(w422) -> ("source"=w420:string)
              n162 = call-poly "CoreLib.data 2 byte array.vi"("string"=w420) -> ("byteArray out"=w421:T4)  [unwired: 18 in]
            }
          }
          n163 = Unbundle By Name(w406) -> ("code"=w409:i32)
          n164 = Bundle By Name(cluster=w398, "Data"=w407, "Error #"=w409, "Data Descriptor"="C:N") -> (w408:T5)
        }
        frame "Set Allow Configure" {
          n165 = Unbundle By Name(w427) -> ("Data"=w431:T4)
          n166 = call-poly "CoreLib.byte array 2 data.vi"("byteArray"=w431) -> ("i16"=w432:i16, "error out"=w430:errorcluster)  [unwired: 16 in, 1 out]
          n167 = Greater Than 0?(x=w432) -> (x > 0?=w424:bool)
          n168 = case shown="No Error" w430 {
            tunnel: [w441 w459] -> w428
            tunnel: w429 -> [w450 w459]
            tunnel: w426 -> [w449 w458]
            tunnel: [w439 w457] -> w425
            tunnel: w423 -> [_ w456]
            tunnel: w424 -> [w448 _]
            frame No Error {
              w443 = u16[] [0, 1, 2, 3] items=["Channel 1", "Channel 2", "Channel 3", "Channel 4", "Math 1", "Math 2", "Math 3", "Math 4", "Reference 1", "Reference 2", "Reference 3", "Reference 4"]
              n169 = call "PH_Tektronix_7000.PC Set Allow Configure.vi"("i ref in"=w450, "Allow Configure?"=w448, "error in (no error)"=w449) -> ("i ref out"=w442:refnum<vi>, "error out"=w440:errorcluster)  [unwired: 15 in]
              n170 = for {
                shift-right: [w452] -> w444
                shift-left: w440 -> [w455]
                shift-right: [w454] -> w445
                shift-left: w442 -> [w453]
                tunnel: w443 -> [w451] mode=indexing
                n171 = call "PH_Tektronix_7000.get Channel Configuration.vi"("i ref in"=w453, "Channel"=w451, "error IO"=w455) -> ("i ref out"=w454:refnum<vi>, "error out"=w452:errorcluster)  [unwired: 15 in]
              }
              n172 = call "PH_Tektronix_7000.get Trigger Configuration.vi"("i ref in"=w445, "error IO"=w444) -> ("i ref out"=w447:refnum<vi>, "error out"=w446:errorcluster)  [unwired: 16 in]
              n173 = call "PH_Tektronix_7000.get Acquisition Configuration.vi"("i ref in"=w447, "error IO"=w446) -> ("i ref out"=w441:refnum<vi>, "error out"=w439:errorcluster)  [unwired: 16 in]
            }
            frame Error {
              n174 = call "CoreLib.set data type mismatch.vi"("error in (no error)"=w458, "error source"=w456) -> ("error out"=w457:errorcluster)  [unwired: 17 in]
            }
          }
          n175 = call "BaseProcess.set event status.vi"("i ref in"=w428, "EventStatus"=w423, "error in (no error)"=w425) -> ("i ref out"=w434:refnum<vi>, "error out"=w435:errorcluster)  [unwired: 14 in, 1 out]
          n176 = case shown="No Error" w435 {
            selector: w435 -> [_ w463]
            tunnel: [T4 [] ("byteArray out") w462] -> w436
            frame No Error {
            }
            frame Error {
              n177 = Unbundle By Name(w463) -> ("source"=w461:string)
              n178 = call-poly "CoreLib.data 2 byte array.vi"("string"=w461) -> ("byteArray out"=w462:T4)  [unwired: 18 in]
            }
          }
          n179 = Unbundle By Name(w435) -> ("code"=w438:i32)
          n180 = Bundle By Name(cluster=w427, "Data"=w436, "Error #"=w438, "Data Descriptor"="C:N") -> (w437:T5)
        }
        frame "Fetch Data before PSDB" {
          n181 = Unbundle By Name(w468) -> ("Data"=w472:T4)
          n182 = call-poly "CoreLib.byte array 2 data.vi"("byteArray"=w472) -> ("i16"=w473:i16, "error out"=w471:errorcluster)  [unwired: 16 in, 1 out]
          n183 = Greater Than 0?(x=w473) -> (x > 0?=w465:bool)
          n184 = case shown="No Error" w471 {
            tunnel: [w481 w488] -> w469
            tunnel: w470 -> [w484 w488]
            tunnel: w467 -> [w483 w487]
            tunnel: [w482 w486] -> w466
            tunnel: w464 -> [_ w485]
            tunnel: w465 -> [w480 _]
            frame No Error {
              n185 = call "PH_Tektronix_7000.PC Fetch Data before sending to PSDB.vi"("i ref in"=w484, "Fetch Data before sending to PSDB?"=w480, "error IO"=w483) -> ("i ref out"=w481:refnum<vi>, "error out"=w482:errorcluster)  [unwired: 15 in]
            }
            frame Error {
              n186 = call "CoreLib.set data type mismatch.vi"("error in (no error)"=w487, "error source"=w485) -> ("error out"=w486:errorcluster)  [unwired: 17 in]
            }
          }
          n187 = call "BaseProcess.set event status.vi"("i ref in"=w469, "EventStatus"=w464, "error in (no error)"=w466) -> ("i ref out"=w475:refnum<vi>, "error out"=w476:errorcluster)  [unwired: 14 in, 1 out]
          n188 = case shown="No Error" w476 {
            selector: w476 -> [_ w492]
            tunnel: [T4 [] ("byteArray out") w491] -> w477
            frame No Error {
            }
            frame Error {
              n189 = Unbundle By Name(w492) -> ("source"=w490:string)
              n190 = call-poly "CoreLib.data 2 byte array.vi"("string"=w490) -> ("byteArray out"=w491:T4)  [unwired: 18 in]
            }
          }
          n191 = Unbundle By Name(w476) -> ("code"=w479:i32)
          n192 = Bundle By Name(cluster=w468, "Data"=w477, "Error #"=w479, "Data Descriptor"="C:N") -> (w478:T5)
        }
        frame "SetPeriodicInterval" {
          n193 = Unbundle By Name(w497) -> ("Data"=w501:T4)
          n194 = call-poly "CoreLib.byte array 2 data.vi"("byteArray"=w501) -> ("i32"=w493:i32, "error out"=w500:errorcluster)  [unwired: 16 in, 1 out]
          n195 = case shown="No Error" w500 {
            tunnel: [w515 w528] -> w498
            tunnel: w499 -> [w519 w528]
            tunnel: w496 -> [w520 w527]
            tunnel: [w517 w526] -> w495
            tunnel: w494 -> [_ w525]
            tunnel: w493 -> [w510 _]
            frame No Error {
              w508 = 100 ("y")
              w513 = -1 ("y")
              n196 = Greater Or Equal?(x=w510, y=w508) -> (x >= y?=w511:bool)
              n197 = Equal?(x=w510, y=w513) -> (x = y?=w514:bool)
              n198 = Select(t=w510, s=w511, f=w508) -> (s? t:f=w509:i32)
              n199 = Select(t=w513, s=w514, f=w509) -> (s? t:f=w512:i32)
              n200 = call "CSSystemLib.ref2name.vi"("obj refnum"=w519) -> ("name"=w521:string)
              n201 = call "BaseProcess.set pdc interval.vi"("i ref in"=w519, "PeriodicInterval [ms]"=w512, "error in (no error)"=w520) -> ("i ref out"=w524:refnum<vi>, "error out"=w523:errorcluster)  [unwired: 14 in, 1 out]
              n202 = call "BaseProcess.call process 2.vi"("i ref in"=w524, "Object"=w521, "Selector"="WakeupPeriodic", "error in (no error)"=w523) -> ("i ref out"=w518:refnum<vi>, "error out"=w516:errorcluster)  [unwired: 14 in]
              n203 = call "PH_Tektronix_7000.get Periodic Interval.vi"("i ref in"=w518, "error in"=w516) -> ("i ref out"=w515:refnum<vi>, "error out"=w517:errorcluster)  [unwired: 16 in]
            }
            frame Error {
              n204 = call "CoreLib.set data type mismatch.vi"("error in (no error)"=w527, "error source"=w525) -> ("error out"=w526:errorcluster)  [unwired: 17 in]
            }
          }
          n205 = call "BaseProcess.set event status.vi"("i ref in"=w498, "EventStatus"=w494, "error in (no error)"=w495) -> ("i ref out"=w503:refnum<vi>, "error out"=w504:errorcluster)  [unwired: 14 in, 1 out]
          n206 = case shown="No Error" w504 {
            selector: w504 -> [_ w532]
            tunnel: [T4 [] ("byteArray out") w531] -> w505
            frame No Error {
            }
            frame Error {
              n207 = Unbundle By Name(w532) -> ("source"=w530:string)
              n208 = call-poly "CoreLib.data 2 byte array.vi"("string"=w530) -> ("byteArray out"=w531:T4)  [unwired: 18 in]
            }
          }
          n209 = Unbundle By Name(w504) -> ("code"=w507:i32)
          n210 = Bundle By Name(cluster=w497, "Data"=w505, "Error #"=w507, "Data Descriptor"="C:N") -> (w506:T5)
        }
        frame "_set_PSDB_Data" {
          n211 = call "CAEObj.unfold trend data.vi"("i ref in"=w537, "raw trend data"=w533) -> ("quality"=w542:i32, "no link"=w539:bool, "data"=w541:i8[], "typeDescriptor"=w540:string, "error out"=w538:errorcluster)  [unwired: 9 in, 4 out]
          n212 = case shown="No Error" w538 {
            tunnel: w536 -> [w556 w593]
            tunnel: [w562 w592] -> w535
            tunnel: [w561 w593] -> w534
            tunnel: w537 -> [w557 w592]
            tunnel: w539 -> [w553 _]
            tunnel: w540 -> [w554 _]
            tunnel: w541 -> [w555 _]
            tunnel: w542 -> [w552 _]
            frame No Error {
              n213 = call "PH_PSDBWriter.get Subsystem DIM Service.vi"("no link"=w553, "typeDescriptor"=w554, "data"=w555, "quality"=w552) -> ("PHELIX Subsystems"=w551:T7)
              n214 = call "PH_PSDBWriter.check PSDB writing condition.vi"("i ref in"=w557, "wanted Subsystem"=w551, "error IO"=w556) -> ("i ref out"=w559:refnum<vi>, "write PSDB?"=w558:bool, "error out"=w560:errorcluster)  [unwired: 14 in]
              n215 = case shown="True" w558 {
                tunnel: w560 -> [w563 w567]
                tunnel: [w564 w570] -> w562
                tunnel: [w563 w569] -> w561
                tunnel: w559 -> [w564 w568]
                frame False {
                }
                frame True {
                  n216 = flat-sequence {
                    tunnel: w567 -> [w572]
                    tunnel: w568 -> [w573]
                    tunnel: [w573] -> w566
                    tunnel: [w572] -> w565
                    tunnel: [w584] -> w570
                    tunnel: [w582] -> w569
                    tunnel: w566 -> [w577]
                    tunnel: w565 -> [w575]
                    frame #0 {
                      n217 = Wait (ms)(milliseconds to wait=u32 5000) -> ()  [unwired: 1 out]
                    }
                    frame #1 {
                      n218 = call "PH_Tektronix_7000.get i attribute.vi"("i ref in"=w577, "error in (no error)"=w575) -> ("i ref out"=w578:refnum<vi>, "i attribute"=w579:T8, "error out"=w580:errorcluster)  [unwired: 15 in]
                      n219 = Unbundle By Name(w579) -> ("Fetch Data before sending to PSDB?"=w581:bool)
                      n220 = case shown="True" w581 {
                        tunnel: w578 -> [w587 w591]
                        tunnel: [w587 w590] -> w576
                        tunnel: w580 -> [w586 w589]
                        tunnel: [w586 w588] -> w574
                        frame False {
                        }
                        frame True {
                          n221 = call "PH_Tektronix_7000.Fetch Waveform.vi"("i ref in"=w591, "error IO"=w589) -> ("i ref out"=w590:refnum<vi>, "error out"=w588:errorcluster)  [unwired: 16 in]
                        }
                      }
                      n222 = call "PH_Tektronix_7000.PC Write PSDB.vi"("i ref in"=w576, "error IO"=w574) -> ("i ref out"=w585:refnum<vi>, "error out"=w583:errorcluster)  [unwired: 16 in]
                      n223 = call "PH_PSDBWriter.evt call write PSDB.vi"("i ref in"=w585, "error in (no error)"=w583) -> ("i ref out"=w584:refnum<vi>, "error out"=w582:errorcluster)  [unwired: 16 in]
                    }
                  }
                }
              }
            }
            frame Error {
            }
          }
          n224 = call "BaseProcess.set event status.vi"("i ref in"=w535, "EventStatus"=w543, "error in (no error)"=w534) -> ("i ref out"=w546:refnum<vi>, "error out"=w547:errorcluster)  [unwired: 14 in, 1 out]
          n225 = case shown="No Error" w547 {
            selector: w547 -> [_ w597]
            tunnel: [T4 [] ("byteArray out") w596] -> w548
            frame No Error {
            }
            frame Error {
              n226 = Unbundle By Name(w597) -> ("source"=w595:string)
              n227 = call-poly "CoreLib.data 2 byte array.vi"("string"=w595) -> ("byteArray out"=w596:T4)  [unwired: 18 in]
            }
          }
          n228 = Unbundle By Name(w547) -> ("code"=w550:i32)
          n229 = Bundle By Name(cluster=w544, "Data"=w548, "Error #"=w550, "Data Descriptor"="C:N") -> (w549:T5)
        }
        frame "Close" {
          n230 = call "PH_Tektronix_7000.Close.vi"("i ref in"=w601, "error in(no error)"=w599) -> ("i ref out"=w600:refnum<vi>, "error out"=w598:errorcluster)  [unwired: 16 in]
          n231 = call "BaseProcess.set event status.vi"("i ref in"=w600, "EventStatus"=w602, "error in (no error)"=w598) -> ("i ref out"=w605:refnum<vi>, "error out"=w606:errorcluster)  [unwired: 14 in, 1 out]
          n232 = case shown="No Error" w606 {
            selector: w606 -> [_ w613]
            tunnel: [T4 [] ("byteArray out") w612] -> w607
            frame No Error {
            }
            frame Error {
              n233 = Unbundle By Name(w613) -> ("source"=w611:string)
              n234 = call-poly "CoreLib.data 2 byte array.vi"("string"=w611) -> ("byteArray out"=w612:T4)  [unwired: 18 in]
            }
          }
          n235 = Unbundle By Name(w606) -> ("code"=w609:i32)
          n236 = Bundle By Name(cluster=w603, "Data"=w607, "Error #"=w609, "Data Descriptor"="C:N") -> (w608:T5)
        }
      }
    }
    frame Error {
    }
  }
  "answer cluster" <- w7
  "i ref out" <- w3
  "error out" <- w2
